vi "Previous Element Sum.vi"() -> ()   [LabVIEW 2025]
panel:
  out "Output Array":dbl[](array[numeric])
  in  "Input Array":dbl[](array[numeric])
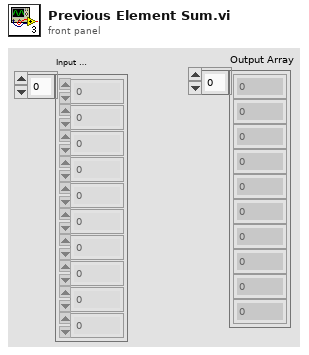
[diagram p1: front panel]
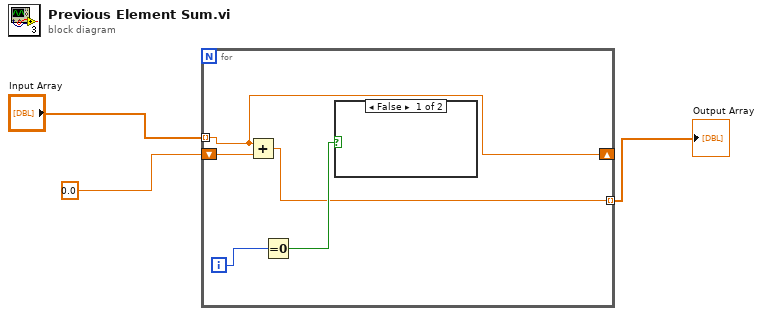
[diagram p0: block diagram]
diagram:
  n1 = for {
    tunnel: "Input Array" -> [w4] mode=indexing
    shift-right: [w4] -> _
    shift-left: 0.0 -> [w5]
    tunnel: [w6] -> w1 mode=indexing
    i -> [w8]
    n2 = Add(x=w4, y=w5) -> (x+y=w6:dbl)
    n3 = Equal To 0?(x=w8) -> (x = 0?=w7:bool)
    n4 = case shown="False" w7 {
      frame False {
      }
      frame True {
      }
    }
  }
  "Output Array" <- w1
